vi "Check Table.vi"(8 "error in (no error)":errorcluster, 11 "Table in":refnum<class "Table.lvclass">) -> (0 "error out":errorcluster, 3 "Table out":refnum<class "Table.lvclass">)   [LabVIEW 2020, in "Table.lvlib" / "Table.lvclass"]
uses:
  Table.lvclass
panel:
  # "Todo: checks that each column of the table is correctly populated\nUse decorator objects to assign PK and FK properties to the columns"
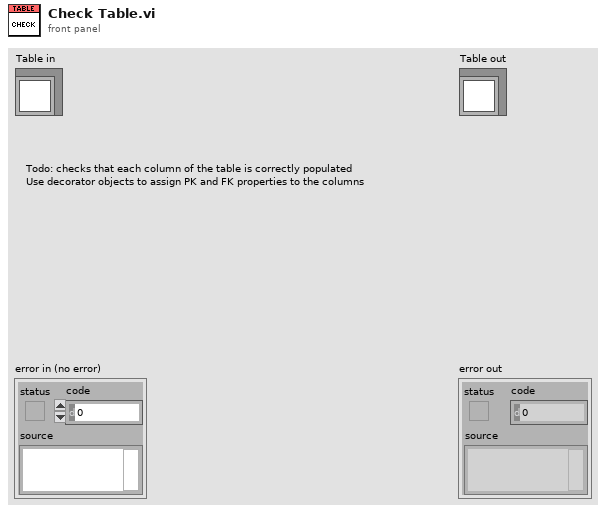
[diagram p1: front panel]
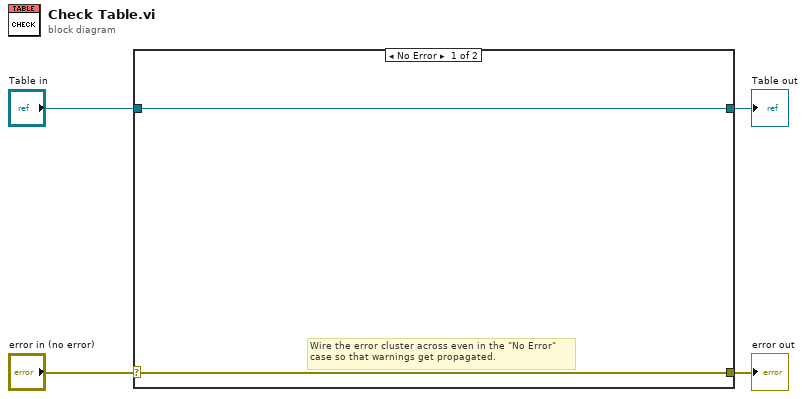
[diagram p0: block diagram]
diagram:
  n1 = case shown="No Error" "error in (no error)" {
    selector: "error in (no error)" -> [w5 w8]
    tunnel: [w5 w8] -> w3
    tunnel: [w6 w7] -> w1
    tunnel: "Table in" -> [w6 w7]
    frame No Error {
      # "Wire the error cluster across even in the \"No Error\"\ncase so that warnings get propagated."
    }
    frame Error {
    }
  }
  "error out" <- w3
  "Table out" <- w1
